vi "Init.vi"(8 "error in (no error)":errorcluster caption="错误输入（无错误）", 10 "size":i32=128, 11 "FIFO(DBL) 输入":refnum<class "FIFO(Boolean).lvclass"> caption="DNL_LabVIEW Object in") -> (0 "error out":errorcluster caption="错误输出", 3 "FIFO(DBL) 输出":refnum<class "FIFO(Boolean).lvclass"> caption="DNL_LabVIEW Object out")   [LabVIEW 2012, in "FIFO(Boolean).lvclass"]
uses:
  FIFO(Boolean).lvclass
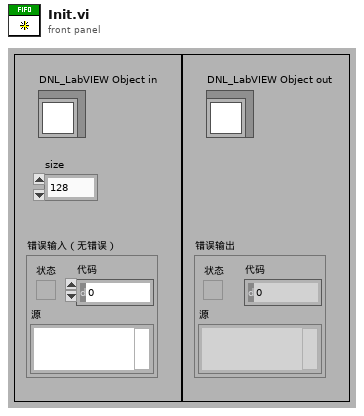
[diagram p1: front panel]
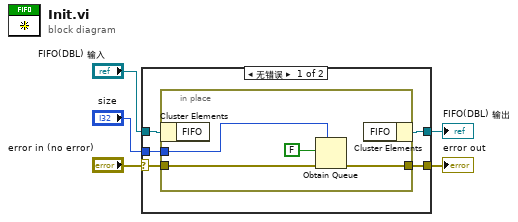
[diagram p0: block diagram]
diagram:
  n1 = case shown="无错误" "error in (no error)" {
    selector: "error in (no error)" -> [w9 w16]
    tunnel: [w8 w16] -> w4
    tunnel: [w7 w15] -> w2
    tunnel: "FIFO(DBL) 输入" -> [w10 w15]
    tunnel: "size" -> [w6 _]
    frame No Error {
      n2 = in-place {
        in-place-border: w9 -> [w14]
        in-place-border: [w13] -> w8
        in-place-border: w6 -> [w12]
        n3 = in-place-cluster #1(w10) -> ()  [unwired: 1 out]
        n4 = Obtain Queue(max queue size (-1, unlimited)=w12, element data type=FALSE, error in (no error)=w14) -> (error out=w13:errorcluster)  [unwired: 2 in, 2 out]
        n5 = in-place-cluster #1() -> (w7:refnum<class "FIFO(Boolean).lvclass">)  [unwired: 1 in]
      }
    }
    frame Error {
    }
  }
  "error out" <- w4
  "FIFO(DBL) 输出" <- w2
